vi "Get Subscribe Data Events.vi"(11 "UserEvents in":refnum<class "User Events.lvclass">) -> (2 "Subscribe Data Events":T1, 3 "UserEvents out":refnum<class "User Events.lvclass">)   [LabVIEW 2016]
uses:
  User Events.lvclass
  Typedefs/Subscribe Data Events.ctl
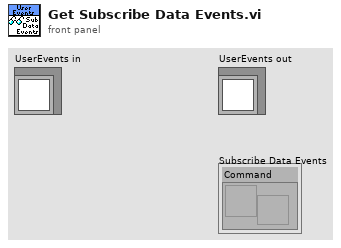
[diagram p1: front panel]
types:
  T1 = typedef "Subscribe Data Events.ctl" = cluster{"Command":refnum<user-event>}
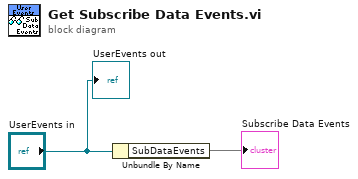
[diagram p0: block diagram]
diagram:
  n1 = Unbundle By Name("UserEvents in") -> ("SubDataEvents"=→"Subscribe Data Events")
  "UserEvents out" <- "UserEvents in"
